vi "Configure Units.vi"(0 "VISA resource name":refnum<visa-resource-name>, 5 "Temperature (0: Celsius)":u16(ring) items=["Celsius", "Fahrenheit", "Kelvins"], 7 "DC Voltage (0: V)":u16(ring) items=["Volts", "dB"], 9 "DC dB Reference Voltage (1 V)":dbl=1.0, 11 "error in (no error)":errorcluster, 12 "AC Voltage (0: V)":u16(ring) items=["Volts", "dB"], 13 "AC dB Reference Voltage (1 V)":dbl=1.0) -> (4 "VISA resource name out":refnum<visa-resource-name>, 15 "error out":errorcluster)   [LabVIEW 2020, in "Keithley 27XX.lvlib"]
doc: "This VI configures the units for temperature measurements. It also provides a method for interpreting Voltage Measurements in dB."
uses:
  Keithley 27XX.lvlib
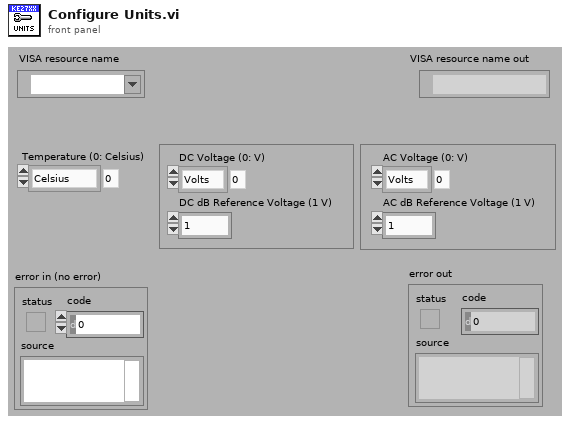
[diagram p1: front panel]
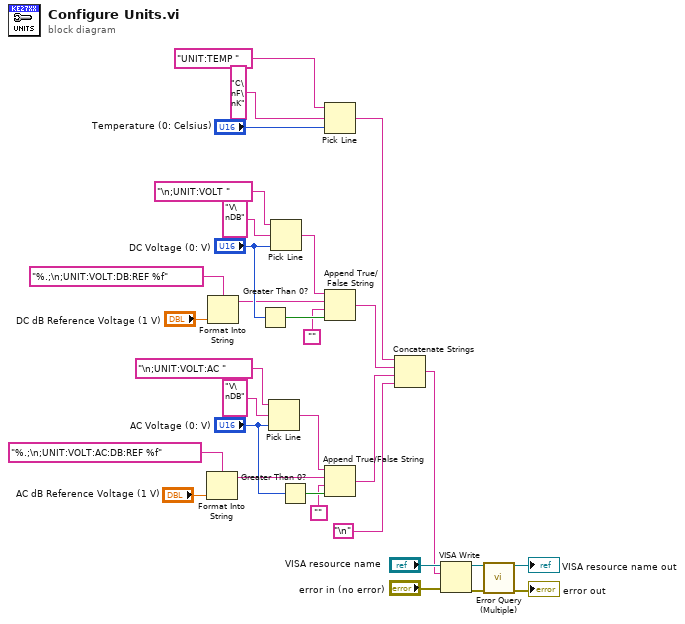
[diagram p0: block diagram]
diagram:
  n1 = Format Into String(format string="%.;\n;UNIT:VOLT:AC:DB:REF %f", "AC dB Reference Voltage (1 V)") -> (resulting string=w7:string)  [unwired: 2 in, 1 out]
  n2 = Format Into String(format string="%.;\n;UNIT:VOLT:DB:REF %f", "DC dB Reference Voltage (1 V)") -> (resulting string=w9:string)  [unwired: 2 in, 1 out]
  n3 = Greater Than 0?(x="DC Voltage (0: V)") -> (x > 0?=w16:bool)
  n4 = Pick Line(string ("")="\n;UNIT:VOLT:AC ", multi-line string="V\nDB", line index="AC Voltage (0: V)") -> (output string=w18:string)
  n5 = Pick Line(string ("")="\n;UNIT:VOLT ", multi-line string="V\nDB", line index="DC Voltage (0: V)") -> (output string=w14:string)
  n6 = Greater Than 0?(x="AC Voltage (0: V)") -> (x > 0?=w21:bool)
  n7 = Pick Line(string ("")="UNIT:TEMP ", multi-line string="C\nF\nK", line index="Temperature (0: Celsius)") -> (output string=w25:string)
  n8 = Append True/False String(1:w16, 2:"", 3:w9, 4:w14) -> (0:w13:string)
  n9 = Append True/False String(1:w21, 2:"", 3:w7, 4:w18) -> (0:w17:string)
  n10 = Concatenate Strings(w25, w13, w17, "\n") -> (w22:string)
  n11 = VISA Write(VISA resource name="VISA resource name", write buffer=w22, error in (no error)="error in (no error)") -> (VISA resource name out=w5:refnum<visa-resource-name>, error out=w4:errorcluster)  [unwired: 1 out]
  n12 = call "Error Query (Multiple).vi"("VISA resource name"=w5, "error in (no error)"=w4) -> ("VISA resource name out"=→"VISA resource name out":refnum<visa-resource-name>, "error out"=→"error out":errorcluster)  [unwired: 10 in, 2 out]
